vi "Configure Volume Resistivity Test.vi"(0 "VISA resource name":refnum<visa-resource-name>, 1 "Volume Pre-discharge Time (10 s)":dbl=10.0, 2 "Volume Measure Time (1 s)":dbl=1.0, 5 "Volume Bias Voltage (500)":dbl=500.0, 7 "Volume Bias Time (1 s)":dbl=1.0, 9 "Volume Discharge Time (2 s)":dbl=2.0, 11 "error in (no error)":errorcluster, 12 "Volume Measure Voltage (500)":dbl=500.0) -> (4 "VISA resource name out":refnum<visa-resource-name>, 15 "error out":errorcluster)   [LabVIEW 2020, in "Keithley 6517.lvlib"]
doc: "Sets the volume resistivity test.\n\nNote:\nCall <b> Configure Test Sequence Common Characteristics </b> first to arm and configures the test sequence.\n\nThis VI is <B>NOT</B> compatible with model <B>6514</B>."
uses:
  <instrlib>/Keithley 6517/Keithley 6517.lvlib
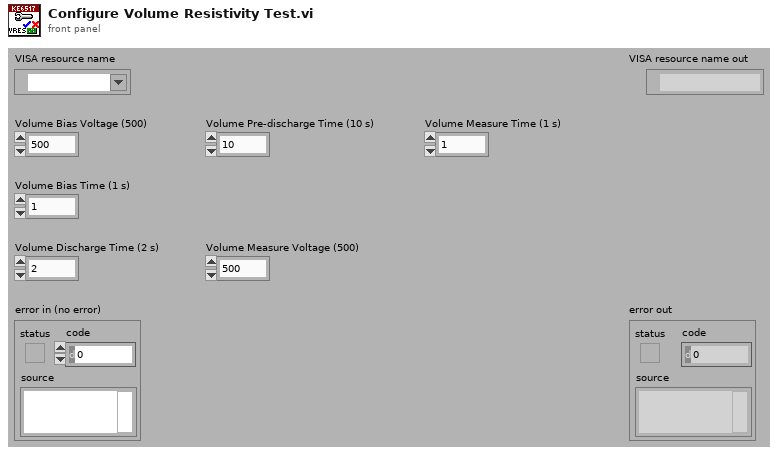
[diagram p1: front panel]
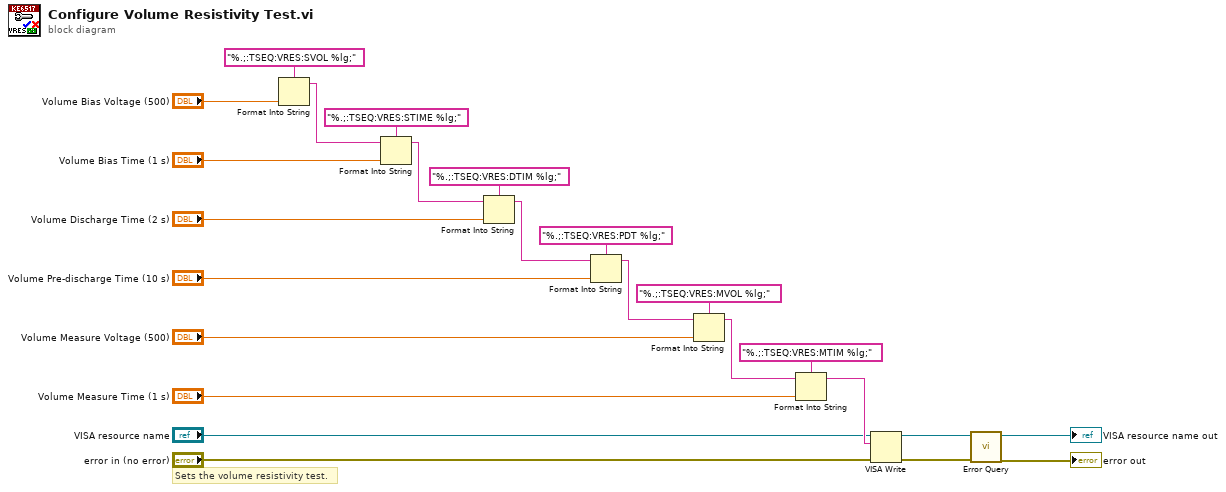
[diagram p0: block diagram]
diagram:
  # "Sets the volume resistivity test."
  n1 = Format Into String(format string="%.;:TSEQ:VRES:SVOL %lg;", "Volume Bias Voltage (500)") -> (resulting string=w22:string)  [unwired: 2 in, 1 out]
  n2 = Format Into String(format string="%.;:TSEQ:VRES:STIME %lg;", initial string=w22, "Volume Bias Time (1 s)") -> (resulting string=w19:string)  [unwired: 1 in, 1 out]
  n3 = Format Into String(format string="%.;:TSEQ:VRES:DTIM %lg;", initial string=w19, "Volume Discharge Time (2 s)") -> (resulting string=w16:string)  [unwired: 1 in, 1 out]
  n4 = Format Into String(format string="%.;:TSEQ:VRES:PDT %lg;", initial string=w16, "Volume Pre-discharge Time (10 s)") -> (resulting string=w13:string)  [unwired: 1 in, 1 out]
  n5 = Format Into String(format string="%.;:TSEQ:VRES:MVOL %lg;", initial string=w13, "Volume Measure Voltage (500)") -> (resulting string=w10:string)  [unwired: 1 in, 1 out]
  n6 = Format Into String(format string="%.;:TSEQ:VRES:MTIM %lg;", initial string=w10, "Volume Measure Time (1 s)") -> (resulting string=w7:string)  [unwired: 1 in, 1 out]
  n7 = VISA Write(VISA resource name="VISA resource name", write buffer=w7, error in (no error)="error in (no error)") -> (VISA resource name out=w4:refnum<visa-resource-name>, error out=w3:errorcluster)  [unwired: 1 out]
  n8 = call <instrlib>:"Error Query.vi"("error in (no error)"=w3, "VISA resource name"=w4) -> ("error out"=→"error out":errorcluster, "VISA resource name out"=→"VISA resource name out":refnum<visa-resource-name>)  [unwired: 6 in, 2 out]
